vi "exp7.vi"() -> ()   [LabVIEW 2019]
uses:
  <vilib>/Analysis/Matrix/Datatypes/RealMatrix.ctl
  <vilib>/Analysis/2dsp.llb/2D Inverse Real FFT.vi
  <vilib>/Analysis/2dsp.llb/2D Real FFT.vi
  <vilib>/Analysis/baseanly.llb/Real Outer Product.vi
  <vilib>/Analysis/2dsp.llb/2D Convolution (DBL).vi
  <vilib>/Analysis/NI_AALBase.lvlib
  <vilib>/Analysis/NI_AALPro.lvlib
  <vilib>/Analysis/Matrix/NI_Matrix.lvlib
panel:
  out "Source Image":u8[][](graph)
  in  "Image Selector":u16(ring) items=["Cameraman", "Couple", "Columbia", "Baboon"]
  out "Filtered Image":dbl[][](graph)
  in  "Stop":bool
  in  "Operator Type":u16(ring) items=["h1", "h2", "Arbitrary"]
  in  "Convolution Mask":T1=[[1.0, 1.0, 1.0], [1.0, -8.0, 1.0], [1.0, 1.0, 1.0]]
  out "Sum":dbl
  out "Inverse Filter Result":dbl[][](graph)
  out "FFT":dbl[][](graph)
  out "Filtered Image FFT":dbl[][](graph)
  in  "ScaleFFTKernel":dbl
  in  "ScaleFilteredImageFFT":dbl
  in  "ScaleInverseFilterResult":dbl
  in  "ScaleFFT":dbl
  out "FFT Kernel":dbl[][](graph)
  in  "ScaleFilteredImage":dbl
  out "Source Image 2":dbl[][](graph)
  in  "Scale New image":dbl
  out "Reconstructed Image":dbl[][](graph)
  in  "Image Selector 2":u16(ring) items=["Cameraman", "Couple", "Columbia", "Baboon", "Ones"]
  in  "Standard Deviation":dbl=1.0000000000000002 format="%0.2f"
  in  "1/SNR":dbl
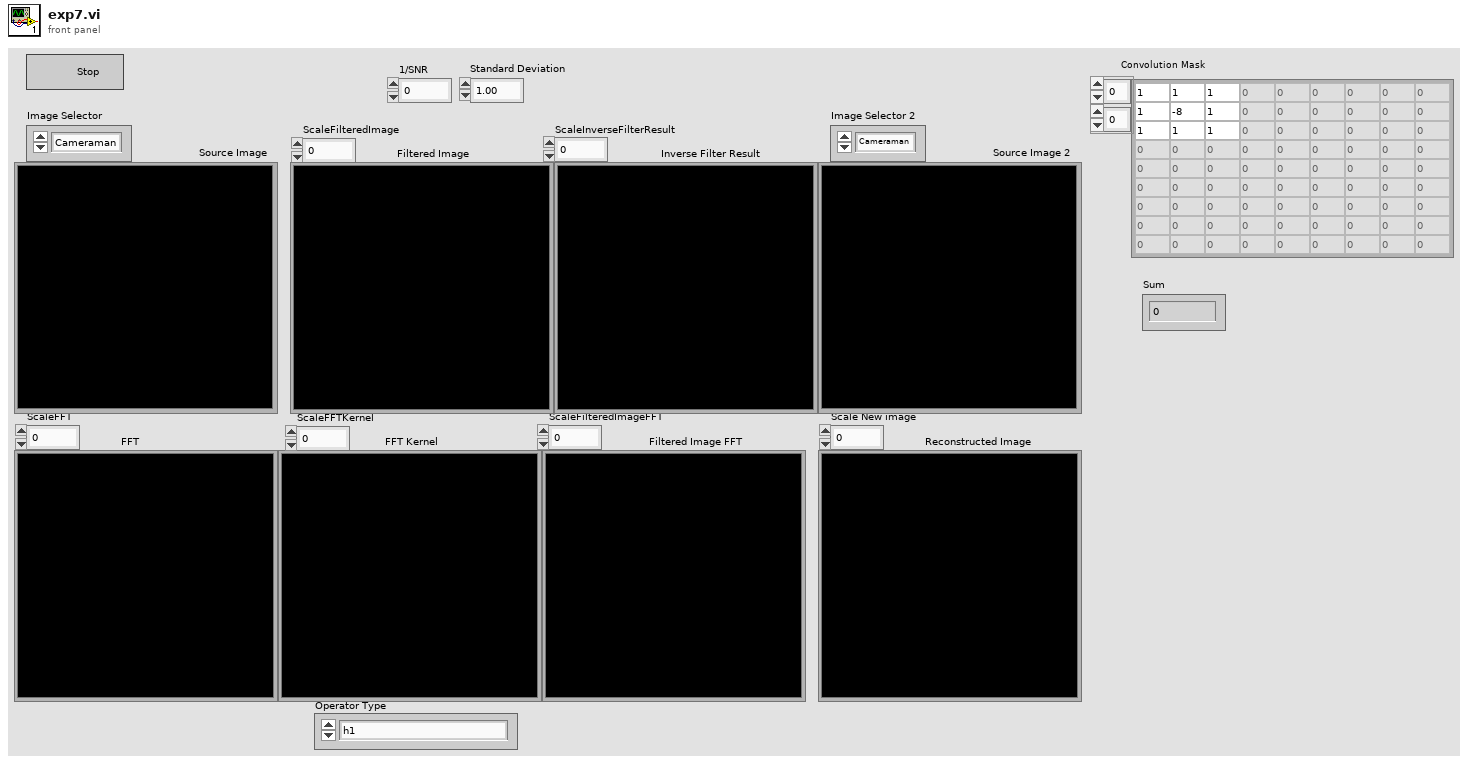
[diagram p1: front panel]
types:
  T1 = typedef "NI_Matrix.lvlib/RealMatrix.ctl" = dbl[][]
  T2 = enum8{"Enabled", "Disabled", "Disabled and Grayed Out"}
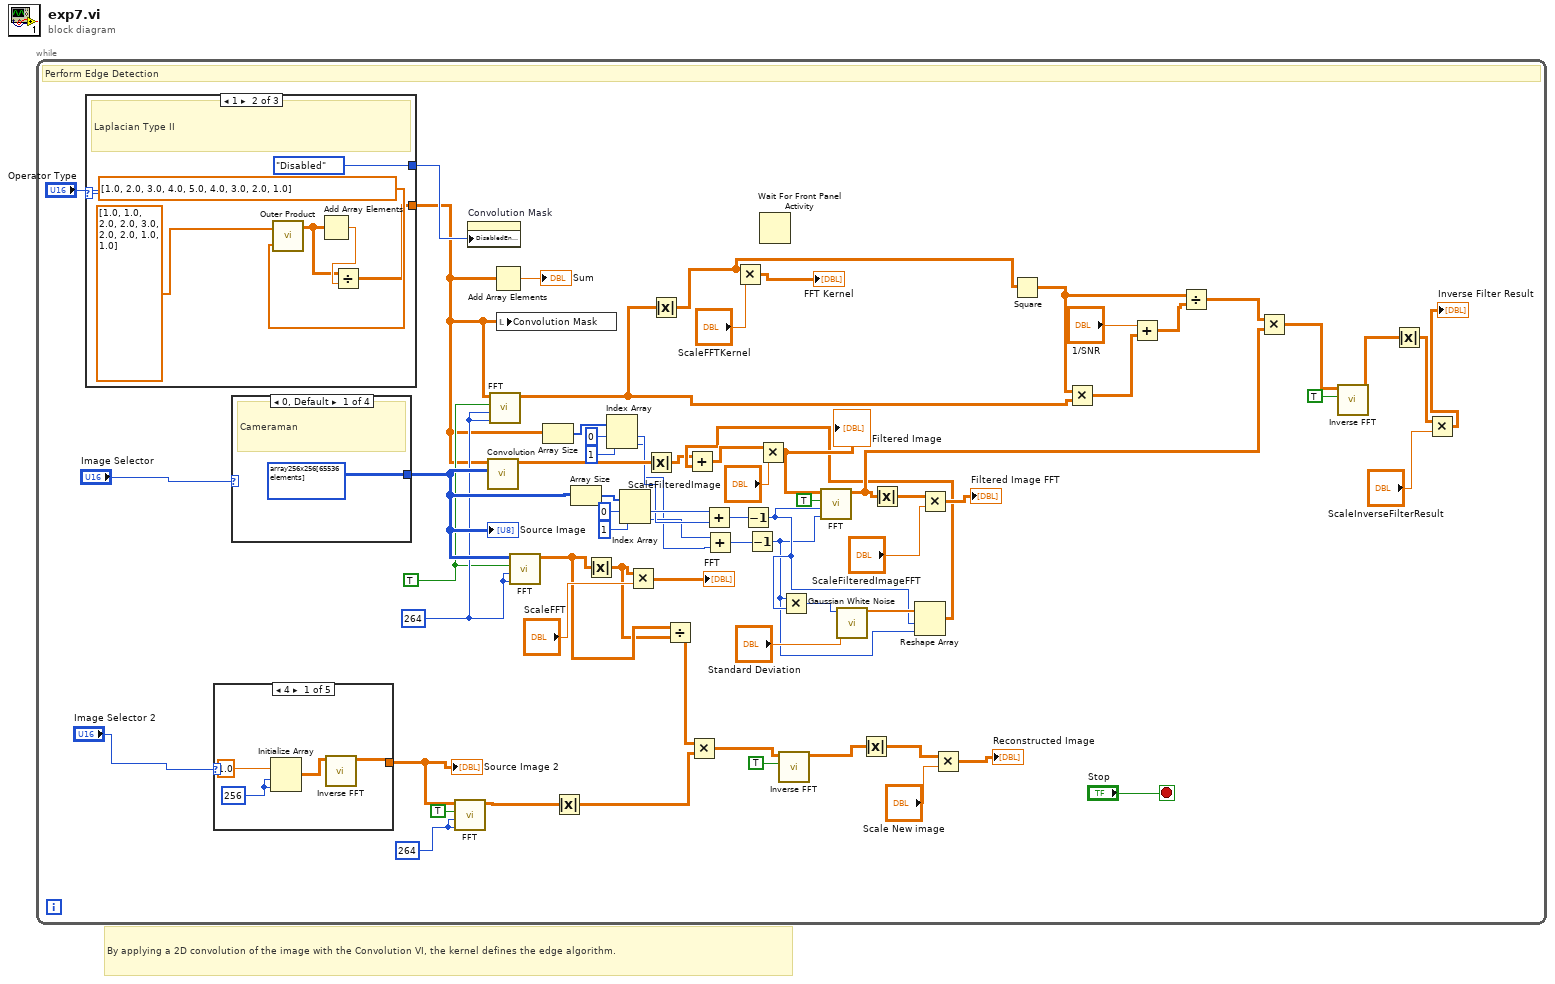
[diagram p0: block diagram]
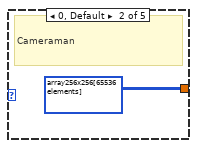
[diagram p2: hidden frame]
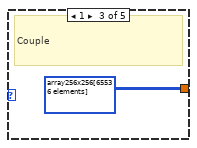
[diagram p3: hidden frame]
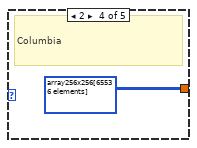
[diagram p4: hidden frame]
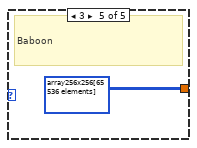
[diagram p5: hidden frame]
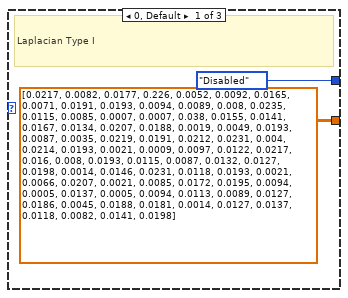
[diagram p6: hidden frame]
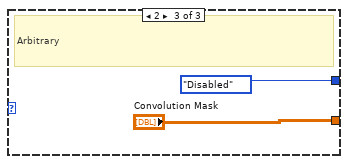
[diagram p7: hidden frame]
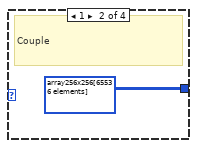
[diagram p8: hidden frame]
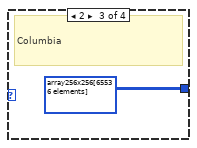
[diagram p9: hidden frame]
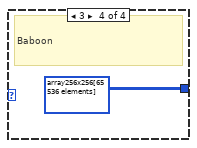
[diagram p10: hidden frame]
diagram:
  # "By applying a 2D convolution of the image with the Convolution VI, the kernel defines the edge algorithm."
  n1 = while {
    stop <- "Stop" stop-if-true
    w39 = 264 ("n")
    w61 = TRUE
    w62 = 264
    # "Perform Edge Detection"
    n2 = case shown="1" "Operator Type" {
      tunnel: [dbl[][] [[0.0217, 0.0082, 0.0177, 0.226, 0.0052, 0.0092, 0.0165, 0.0071, 0.0191], [0.0193, 0.0094, 0.0089, 0.008, 0.0235, 0.0115, 0.0085, 0.0007, 0.0007], [0.038, 0.0155, 0.0141, 0.0167, 0.0134, 0.0207, 0.0188, 0.0019, 0.0049], [0.0193, 0.0087, 0.0035, 0.0219, 0.0191, 0.0212, 0.0231, 0.004, 0.0214], [0.0193, 0.0021, 0.0009, 0.0097, 0.0122, 0.0217, 0.016, 0.008, 0.0193], [0.0115, 0.0087, 0.0132, 0.0127, 0.0198, 0.0014, 0.0146, 0.0231, 0.0118], [0.0193, 0.0021, 0.0066, 0.0207, 0.0021, 0.0085, 0.0172, 0.0195, 0.0094], [0.0005, 0.0137, 0.0005, 0.0094, 0.0113, 0.0089, 0.0127, 0.0186, 0.0045], [0.0188, 0.0181, 0.0014, 0.0127, 0.0137, 0.0118, 0.0082, 0.0141, 0.0198]] w80 "Convolution Mask"] -> w2
      tunnel: [T2."Disabled" ("Disabled") T2."Disabled" ("Disabled") T2."Disabled" ("Disabled")] -> w64
      frame 0, Default {
        # "Laplacian Type I"
      }
      frame 1 {
        # "Laplacian Type II"
        n3 = call-poly <vilib>:"Outer Product.vi"("Y Vector"=dbl[] [1.0, 2.0, 3.0, 4.0, 5.0, 4.0, 3.0, 2.0, 1.0], "X Vector"=dbl[] [1.0, 1.0, 2.0, 2.0, 3.0, 2.0, 2.0, 1.0, 1.0]) -> ("Outer Product"=w81:T1)  [unwired: 1 out]
        n4 = Add Array Elements(numeric array=w81) -> (sum=w82:dbl)
        n5 = Divide(x=w81, y=w82) -> (x/y=w80:T1)
      }
      frame 2 {
        # "Arbitrary"
      }
    }
    n6 = case shown="4" "Image Selector 2" {
      tunnel: [w70 u8[][] array256x256[65536 elements] ("Image Pixels (U8)") u8[][] array256x256[65536 elements] ("Image Pixels (U8)") u8[][] array256x256[65536 elements] ("Image Pixels (U8)") u8[][] array256x256[65536 elements] ("Image Pixels (U8)")] -> w40
      frame 4 {
        w73 = 256 ("dimension size")
        n7 = Initialize Array(1.0, w73, w73) -> (w71:dbl[][])
        n8 = call-poly <vilib>:"Inverse FFT.vi"("FFT {X}"=w71) -> ("X"=w70:dbl[][])  [unwired: 9 in, 1 out]
      }
      frame 0, Default {
        # "Cameraman"
      }
      frame 1 {
        # "Couple"
      }
      frame 2 {
        # "Columbia"
      }
      frame 3 {
        # "Baboon"
      }
    }
    "Source Image 2" <- w40
    n9 = case shown="0, Default" "Image Selector" {
      tunnel: [u8[][] array256x256[65536 elements] ("Image Pixels (U8)") u8[][] array256x256[65536 elements] ("Image Pixels (U8)") u8[][] array256x256[65536 elements] ("Image Pixels (U8)") u8[][] array256x256[65536 elements] ("Image Pixels (U8)")] -> w63
      frame 0, Default {
        # "Cameraman"
      }
      frame 1 {
        # "Couple"
      }
      frame 2 {
        # "Columbia"
      }
      frame 3 {
        # "Baboon"
      }
    }
    "Source Image" <- w63
    n10 = call-poly <vilib>:"FFT.vi"("n"=w39, "m"=w39, "shift?"=TRUE, "X"=w40) -> ("FFT {X}"=w37:cdb[][])  [unwired: 6 in, 1 out]
    n11 = property on="Convolution Mask" class="Arr (strict)"("DisabledEnum"=w64) -> ()  [unwired: 2 in, 2 out]
    n12 = call-poly <vilib>:"Convolution.vi"("Y"=w63, "X"=w2) -> ("X * Y"=w68:dbl[][])  [unwired: 8 in, 1 out]
    n13 = call-poly <vilib>:"FFT.vi"("n"=w62, "m"=w62, "shift?"=w61, "X"=w2) -> ("FFT {X}"=w24:cdb[][])  [unwired: 6 in, 1 out]
    n14 = Add Array Elements(numeric array=w2) -> (sum=→"Sum":dbl)
    n15 = local write "Convolution Mask"(w2) -> ()
    n16 = call-poly <vilib>:"FFT.vi"("n"=w62, "m"=w62, "shift?"=w61, "X"=w63) -> ("FFT {X}"=w35:cdb[][])  [unwired: 6 in, 1 out]
    n17 = Array Size(array=w2) -> (size(s)=w50:i32[])
    n18 = Absolute Value(x=w37) -> (abs(x)=w36:dbl[][])
    n19 = Array Size(array=w63) -> (size(s)=w51:i32[])
    n20 = Absolute Value(x=w35) -> (abs(x)=w34:dbl[][])
    n21 = Index Array(array=w50, index #1=0 ("index"), index #2=1 ("index")) -> (element #1=w46:i32, element #2=w44:i32)
    n22 = Index Array(array=w51, index #1=0 ("index"), index #2=1 ("index")) -> (element #1=w47:i32, element #2=w45:i32)
    n23 = Multiply(x=w34, y="ScaleFFT") -> (x*y=→"FFT":dbl[][])
    n24 = Absolute Value(x=w68) -> (abs(x)=w3:dbl[][])
    n25 = Absolute Value(x=w24) -> (abs(x)=w25:dbl[][])
    n26 = Divide(x=w35, y=w34) -> (x/y=w33:cdb[][])
    n27 = Multiply(x=w33, y=w36) -> (x*y=w32:cdb[][])
    n28 = Add(x=w47, y=w46) -> (x+y=w42:i32)
    n29 = Add(x=w45, y=w44) -> (x+y=w43:i32)
    n30 = Multiply(x=w25, y="ScaleFFTKernel") -> (x*y=→"FFT Kernel":dbl[][])
    n31 = Decrement(x=w42) -> (x-1=w6:i32)
    n32 = Decrement(x=w43) -> (x-1=w5:i32)
    n33 = Wait For Front Panel Activity() -> ()  [unwired: 3 in, 1 out]
    n34 = call-poly <vilib>:"Inverse FFT.vi"("shift?"=TRUE, "FFT {X}"=w32) -> ("X"=w30:dbl[][])  [unwired: 8 in, 1 out]
    n35 = Multiply(x=w5, y=w6) -> (x*y=w9:i32)
    n36 = call <vilib>:"Gaussian White Noise.vi"("standard deviation"="Standard Deviation", "samples"=w9) -> ("Gaussian noise pattern"=w7:dbl[])  [unwired: 8 in, 1 out]
    n37 = Absolute Value(x=w30) -> (abs(x)=w28:dbl[][])
    n38 = Reshape Array(w7, w6, w5) -> (w4:dbl[][])
    n39 = Add(x=w3, y=w4) -> (x+y=w10:dbl[][])
    n40 = Multiply(x=w10, y="ScaleFilteredImage") -> (x*y=w20:dbl[][])
    "Filtered Image" <- w20
    n41 = call-poly <vilib>:"FFT.vi"("n"=w5, "m"=w6, "shift?"=TRUE, "X"=w20) -> ("FFT {X}"=w19:cdb[][])  [unwired: 6 in, 1 out]
    n42 = Absolute Value(x=w19) -> (abs(x)=w56:dbl[][])
    n43 = Multiply(x=w56, y="ScaleFilteredImageFFT") -> (x*y=→"Filtered Image FFT":dbl[][])
    n44 = Multiply(x=w28, y="Scale New image") -> (x*y=→"Reconstructed Image":dbl[][])
    n45 = Square(x=w25) -> (x^2=w21:dbl[][])
    n46 = Multiply(x=w21, y=w24) -> (x*y=w23:cdb[][])
    n47 = Add(x="1/SNR", y=w23) -> (x+y=w22:cdb[][])
    n48 = Divide(x=w21, y=w22) -> (x/y=w18:cdb[][])
    n49 = Multiply(x=w18, y=w19) -> (x*y=w17:cdb[][])
    n50 = call-poly <vilib>:"Inverse FFT.vi"("shift?"=TRUE, "FFT {X}"=w17) -> ("X"=w15:dbl[][])  [unwired: 8 in, 1 out]
    n51 = Absolute Value(x=w15) -> (abs(x)=w13:dbl[][])
    n52 = Multiply(x=w13, y="ScaleInverseFilterResult") -> (x*y=→"Inverse Filter Result":dbl[][])
  }
